vi "Read Plugin Selector.vi"(8 "error in (no error)":errorcluster, 11 "CIF_UI in":refnum<class "CIF_Manager_UI.lvclass">) -> (0 "error out":errorcluster, 3 "Plugin Info":T1 {"Plugin Info"."Node Status"."Monitor Doubles"."4" format="%#_9g"; "Plugin Info"."Node Status"."Monitor Doubles"."3" format="%#_9g"; "Plugin Info"."Node Status"."Monitor Doubles"."2" format="%#_9g"; "Plugin Info"."Node Status"."Monitor Doubles"."1" format="%#_9g"; "Plugin Info"."Node Status"."Timing Statistics (us)"."Period"."Avg" format="%_6g"})   [LabVIEW 2021, in "CIF_Manager_UI.lvclass"]
uses:
  CIF_Manager_UI.lvclass
  C:/Program Files/National Instruments/LabVIEW 2021/vi.lib/CIF Foundation/CIF Core/CIFUI/CIF_UI.lvclass
  <vilib>/CIF Foundation/CIF Core/CIFUI/Typedef/Plugin Connections.ctl
  <vilib>/gRPC/LabVIEW gRPC Library/Shared/grpcId.ctl
  <vilib>/CIF Foundation/CIF Core/CIFCore/Common/Typedef/PluginInfo.ctl
  <vilib>/CIF Foundation/CIF Core/CIFCore/Common/Typedef/Version Simple.ctl
  <vilib>/CIF Foundation/CIF Core/CIFCore/Common/Typedef/gRPC Reported Plugin Status.ctl
  <vilib>/CIF Foundation/CIF Core/CIFCore/Common/Typedef/Plugin State.ctl
  <vilib>/CIF Foundation/CIF Core/CIFCore/Common/Typedef/Timing Statistics.ctl
  <vilib>/CIF Foundation/CIF Core/CIFCore/Common/Typedef/Timing Stats Base.ctl
  <vilib>/CIF Foundation/CIF Core/CIFCore/Common/Typedef/FIFO Statistics.ctl
  <vilib>/CIF Foundation/CIF Core/CIFCore/Common/Typedef/Simple Error.ctl
  <vilib>/CIF Foundation/CIF Core/CIFCore/Common/Typedef/Monitor Doubles.ctl
  <vilib>/CIF Foundation/CIF Core/CIFCore/Common/Typedef/Monitor U64.ctl
  <vilib>/CIF Foundation/CIF Core/CIFCore/Common/Typedef/Monitor I64.ctl
  CIF_Manager_UI.lvclass/CIF_Manager_UI.ctl
  <vilib>/CIF Foundation/CIF Core/CIFUI/CIF_UI.lvclass/CIF_UI.ctl
  <vilib>/CIF Foundation/CIF Core/CIFUI/Accessors/Read Plugin Connection Map.vi
  <vilib>/gRPC/LabVIEW gRPC Library/grpc-lvsupport-release.lvlib
  <vilib>/CIF Foundation/CIF Core/CIFCore/Common/CIFCoreCommon.lvlib
  <vilib>/CIF Foundation/CIF Core/CIFUI/CIF_UI.lvclass
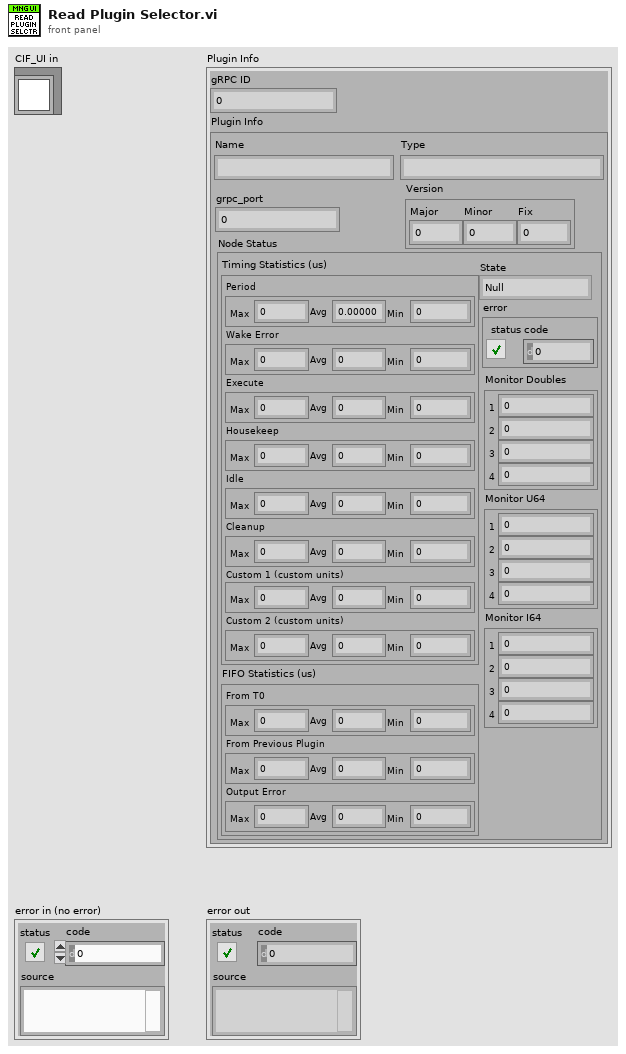
[diagram p1: front panel]
types:
  T1 = typedef "CIF_UI.lvclass/Plugin Connections.ctl" = cluster{"gRPC ID":T2, "Plugin Info":T3}
  T2 = typedef "grpc-lvsupport-release.lvlib/grpcId.ctl" = u64
  T3 = typedef "CIFCoreCommon.lvlib/PluginInfo.ctl" = cluster{"Name":string, "Type":string, "grpc_port":i32, "Version":T4, "Node Status":T5}
  T4 = typedef "CIFCoreCommon.lvlib/Version Simple.ctl" = cluster{"Major":i32, "Minor":i32, "Fix":i32}
  T5 = typedef "CIFCoreCommon.lvlib/gRPC Reported Plugin Status.ctl" = cluster{"State":T6, "Timing Statistics (us)":T7, "FIFO Statistics (us)":T9, "error":T10, "Monitor Doubles":T11, "Monitor U64":T12, "Monitor I64":T13}
  T6 = typedef "CIFCoreCommon.lvlib/Plugin State.ctl" = enum32{"Null", "Creating", "Listening", "Running", "CleaningUp", "Destroying"}
  T7 = typedef "CIFCoreCommon.lvlib/Timing Statistics.ctl" = cluster{"Period":T8, "Wake Error":T8, "Execute":T8, "Housekeep":T8, "Idle":T8, "Cleanup":T8, "Custom 1 (custom units)":T8, "Custom 2 (custom units)":T8}
  T8 = typedef "CIFCoreCommon.lvlib/Timing Stats Base.ctl" = cluster{"Max":i64, "Avg":dbl, "Min":i64}
  T9 = typedef "CIFCoreCommon.lvlib/FIFO Statistics.ctl" = cluster{"From T0":T8, "From Previous Plugin":T8, "Output Error":T8}
  T10 = typedef "CIFCoreCommon.lvlib/Simple Error.ctl" = cluster{"status":bool, "code":i32}
  T11 = typedef "CIFCoreCommon.lvlib/Monitor Doubles.ctl" = cluster{"1":dbl, "2":dbl, "3":dbl, "4":dbl}
  T12 = typedef "CIFCoreCommon.lvlib/Monitor U64.ctl" = cluster{"1":u64, "2":u64, "3":u64, "4":u64}
  T13 = typedef "CIFCoreCommon.lvlib/Monitor I64.ctl" = cluster{"1":i64, "2":i64, "3":i64, "4":i64}
  T14 = typedef "CIF_UI.lvclass/Plugin Connection Map.ctl" = map{string, T1}
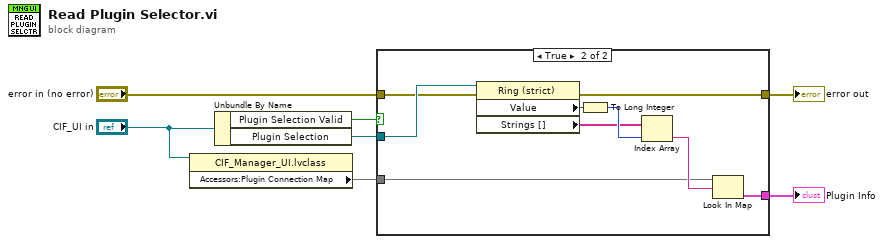
[diagram p0: block diagram]
diagram:
  n1 = property class="CIF_Manager_UI.lvclass"(reference="CIF_UI in") -> ("Accessors:Plugin Connection Map"=w1:T14)  [unwired: 1 in, 2 out]
  n2 = Unbundle By Name("CIF_UI in") -> ("Plugin Selection Valid"=w7:bool, "Plugin Selection"=w6:refnum<vi>)
  n3 = case shown="True" w7 {
    tunnel: w1 -> [_ w14]
    tunnel: w6 -> [_ w15]
    tunnel: "error in (no error)" -> [w8 w13]
    tunnel: [w8 w12] -> w4
    tunnel: [_ w9] -> w3
    frame False {
    }
    frame True {
      n4 = property class="Ring (strict)"(reference=w15, error in=w13) -> (error out=w12:errorcluster, "Value"=w17:u16, "Strings []"=w10:string[])  [unwired: 1 out]
      n5 = To Long Integer(number=w17) -> (32bit integer=w11:i32)
      n6 = Index Array(array=w10, index=w11) -> (element=w16:string)
      n7 = Look In Map(map=w14, key=w16) -> (value=w9:T1)  [unwired: 1 in, 1 out]
    }
  }
  "error out" <- w4
  "Plugin Info" <- w3
